vi "Comunicacion_Arcduino_buck.vi"() -> ()   [LabVIEW 2014]
panel:
  in  "Set Point":dbl(slide) scale=0.0..4.8
  in  "Constante Proporcional":dbl(knob) scale=0.0..10.0
  out "Voltaje de Salida":dynamicdata(graph)
  in  "VISA resource name":refnum<visa-resource-name>
  in  "stop":bool
  in  "Velocidad de Conexion":enum16{"115200", "9600"}(ring)
  in  "error in (no error)":errorcluster
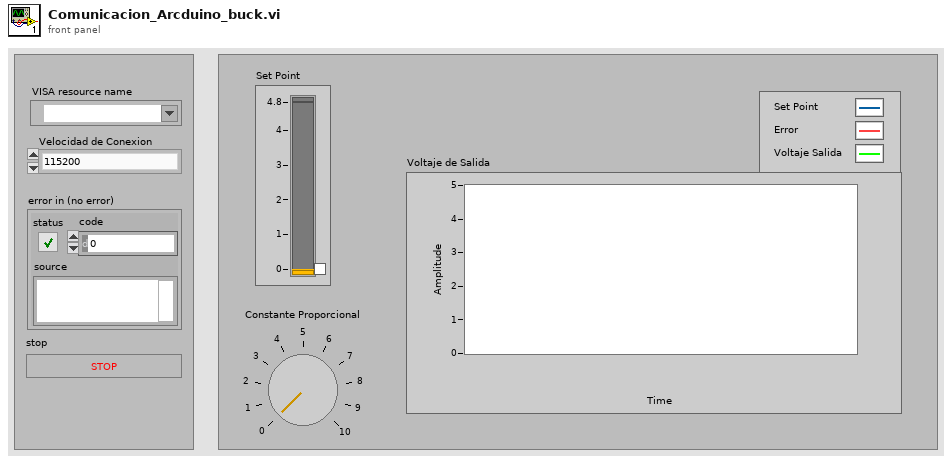
[diagram p1: front panel]
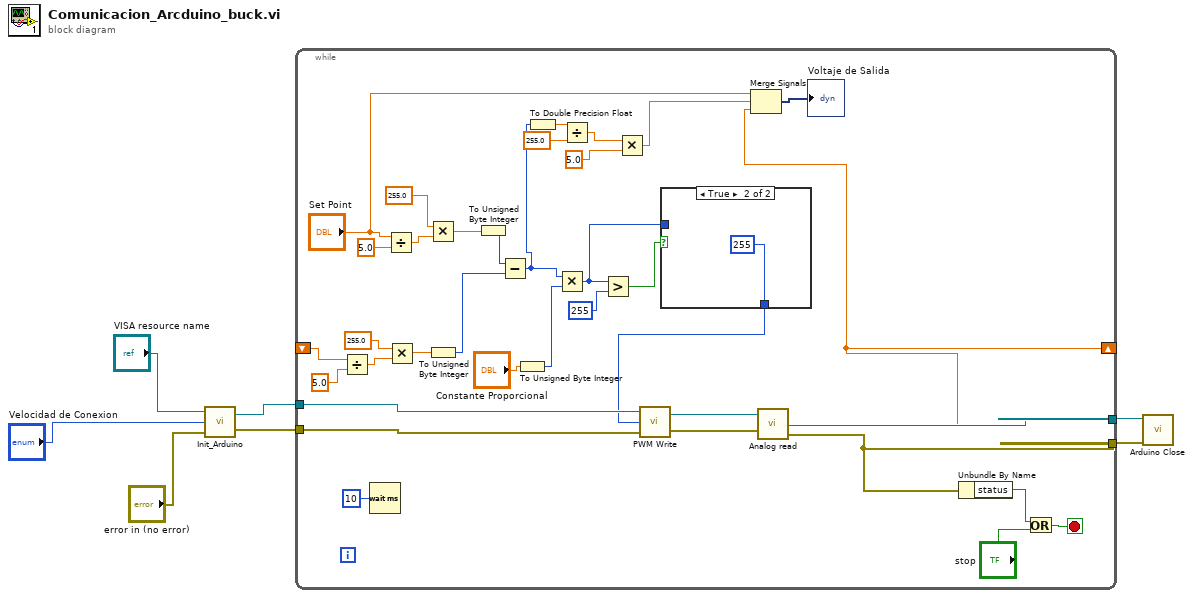
[diagram p0: block diagram]
diagram:
  n1 = call "Init_Arduino.vi"("error in (no error)"="error in (no error)", "Velocidad de Conexion"="Velocidad de Conexion", "VISA Refnum in"="VISA resource name") -> ("error out"=w3:errorcluster, "VISA Refnum out"=w5:refnum<visa-resource-name>)
  n2 = while {
    tunnel: w3 -> [w42]
    tunnel: w5 -> [w43]
    tunnel: [w35] -> w1
    tunnel: [w36] -> w2
    shift-right: [w9] -> _
    shift-left: _ -> [w8]
    stop <- w39 stop-if-true
    n3 = Divide(x=w8, y=5.0) -> (x/y=w33:dbl)
    n4 = Wait (ms)(milliseconds to wait=u32 10) -> ()  [unwired: 1 out]
    n5 = Divide(x="Set Point", y=5.0) -> (x/y=w29:dbl)
    n6 = Multiply(x=255.0, y=w33) -> (x*y=w31:dbl)
    n7 = Multiply(x=255.0, y=w29) -> (x*y=w11:dbl)
    n8 = To Unsigned Byte Integer(number=w31) -> (unsigned 8bit integer=w26:u8)
    n9 = To Unsigned Byte Integer(number=w11) -> (unsigned 8bit integer=w27:u8)
    n10 = Subtract(x=w27, y=w26) -> (x-y=w17:u8)
    n11 = To Unsigned Byte Integer(number="Constante Proporcional") -> (unsigned 8bit integer=w24:u8)
    n12 = To Double Precision Float(number=w17) -> (double precision float=w16:dbl)
    n13 = Multiply(x=w17, y=w24) -> (x*y=w19:u8)
    n14 = Divide(x=w16, y=255.0) -> (x/y=w14:dbl)
    n15 = Greater?(x=w19, y=u8 255) -> (0:w22:bool)
    n16 = Multiply(x=w14, y=5.0) -> (x*y=w12:dbl)
    n17 = case shown="True" w22 {
      tunnel: w19 -> [w44 _]
      tunnel: [w44 u8 255] -> w21
      frame False {
      }
      frame True {
      }
    }
    n18 = call "PWM Write.vi"("error in (no error)"=w42, "Ciclo de Trabajo"=w21, "VISA Refnum in"=w43) -> ("error out"=w37:errorcluster, "VISA Refnum out"=w38:refnum<visa-resource-name>)
    n19 = call "Analog read.vi"("VISA Refnum in"=w38, "error in (no error)"=w37) -> ("VISA Refnum out"=w35:refnum<visa-resource-name>, "Numeric"=w9:dbl, "error out"=w36:errorcluster)
    n20 = Merge Signals("Set Point", w12, w9) -> (→"Voltaje de Salida":dynamicdata)
    n21 = Unbundle By Name(w36) -> ("status"=w41:bool)
    n22 = Or(x=w41, y="stop") -> (x .or. y?=w39:bool)
  }
  n23 = call "Arduino Close.vi"("error in (no error)"=w2, "VISA Refnum in"=w1) -> ()  [unwired: 10 in]
